vi "2020 primative.vi"() -> ()   [LabVIEW 2020]
panel:
  out "delimited string":string
  out "data":string[][](array[string])
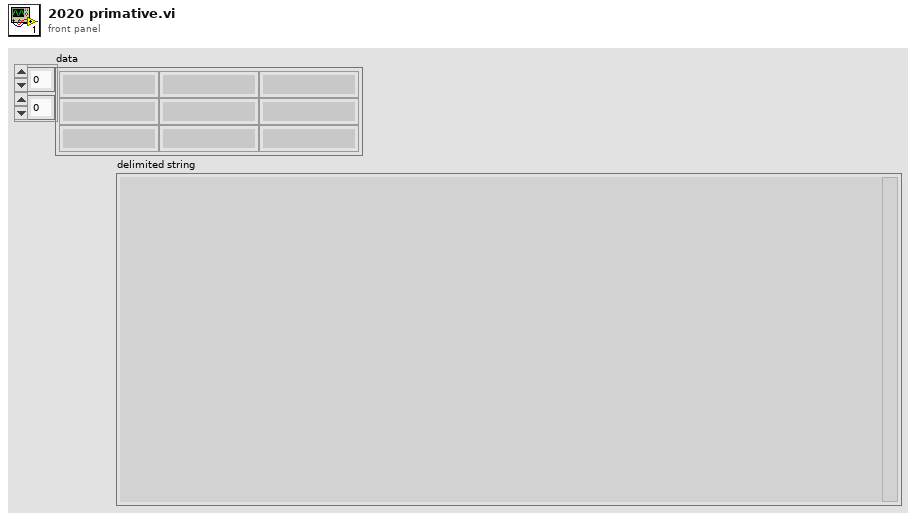
[diagram p1: front panel]
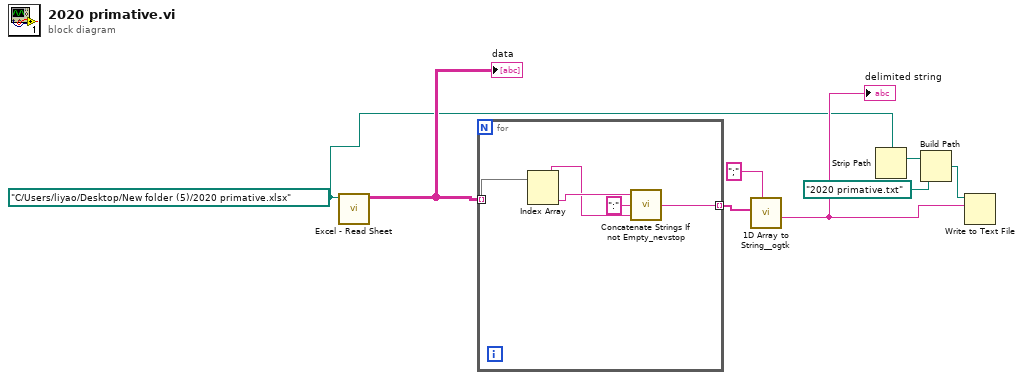
[diagram p0: block diagram]
diagram:
  w4 = path "C:/Users/liyao/Desktop/New folder (5)/2020 primative.xlsx" ("path")
  n1 = call <userlib>:"Excel - Read Sheet.vi"("path"=w4) -> ("data"=w8:string[][])  [unwired: 9 in, 1 out]
  "data" <- w8
  n2 = for {
    tunnel: w8 -> [w13] mode=indexing
    tunnel: [w9] -> w7 mode=indexing
    n3 = Index Array(array=w13) -> (element #1=w11:string, element #2=w12:string)  [unwired: 2 in]
    n4 = call <userlib>:"Concatenate Strings If not Empty_nevstop.vi"("String"=w11, "seperator(:)"=":", "prefix"=w12) -> ("result"=w9:string)  [unwired: 2 in]
  }
  n5 = call <userlib>:"1D Array to String__ogtk.vi"("delimiter (Tab)"=";", "Array of Strings"=w7) -> ("delimited string"=w5:string)  [unwired: 9 in]
  "delimited string" <- w5
  n6 = Strip Path(path=w4) -> (stripped path=w3:path)  [unwired: 1 out]
  n7 = Build Path(base path=w3, name or relative path=path "2020 primative.txt") -> (appended path=w2:path)
  n8 = Write to Text File(file (use dialog)=w2, text=w5) -> ()  [unwired: 2 in, 3 out]
